vi "Set Splash Screen.vi"(8 "error in (no error)":errorcluster, 10 "Splash Screen":refnum<class "Splash Screen.lvclass">, 11 "Volatus Core in":refnum<class "Volatus Core.lvclass">) -> (0 "error out":errorcluster, 3 "Volatus Core out":refnum<class "Volatus Core.lvclass">)   [LabVIEW 2020, in "Volatus.lvlib" / "Volatus Core.lvclass"]
uses:
  Volatus Core.lvclass
  Splash Screen/Splash Screen.lvclass
  Volatus Core.lvclass/Volatus Core.ctl
  Plugin Splash/Plugin Splash.lvclass
  C:/dev/lv20CE/relink/lv-volatus/Volatus/Plugin Splash/Plugin Splash.lvclass
  C:/dev/lv20CE/relink/lv-volatus/Volatus/Splash Screen/Splash Screen.lvclass
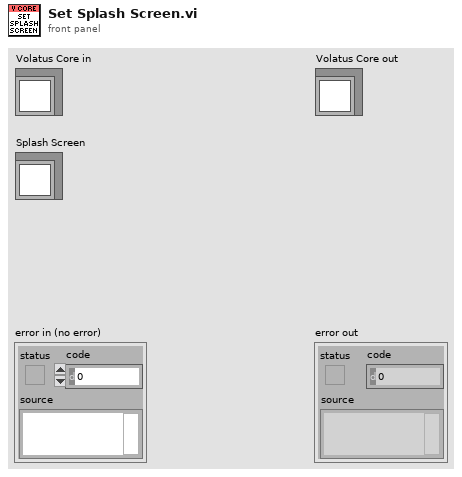
[diagram p1: front panel]
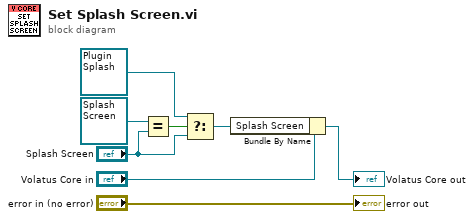
[diagram p0: block diagram]
diagram:
  n1 = Equal?(x=refnum<class "Splash Screen.lvclass"> refnum, y="Splash Screen") -> (x = y?=w5:bool)
  n2 = Select(t=refnum<class "Plugin Splash.lvclass"> refnum ("Volatus:Plugin Splash.lvclass"), s=w5, f="Splash Screen") -> (s? t:f=w1:refnum<class "Splash Screen.lvclass">)
  n3 = Bundle By Name(cluster="Volatus Core in", "Splash Screen"=w1) -> (→"Volatus Core out":refnum<class "Volatus Core.lvclass">)
  "error out" <- "error in (no error)"
